vi "Chart with date and time.vi"(11 "Data in":dbl) -> (3 "Waveform Chart":waveform(dbl)(graph))   [LabVIEW 2018]
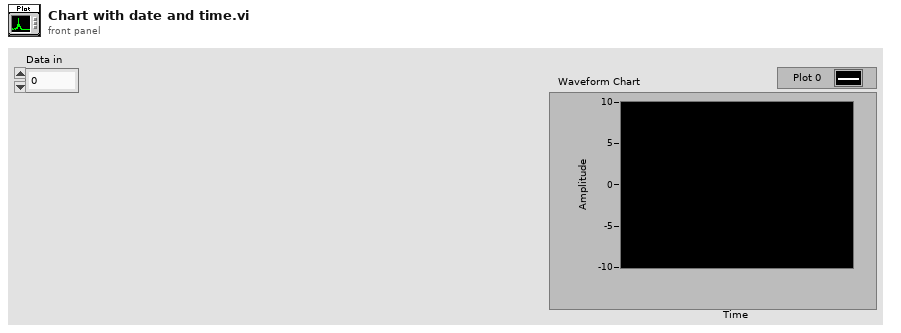
[diagram p1: front panel]
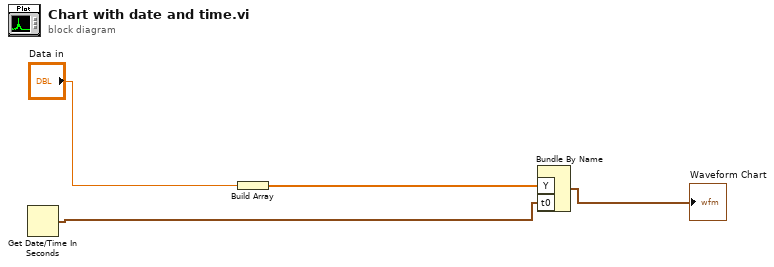
[diagram p0: block diagram]
diagram:
  n1 = Get Date/Time In Seconds() -> (seconds since 1Jan1904=w1:timestamp)
  n2 = Build Array("Data in") -> (w3:dbl[])
  n3 = Bundle By Name("Y"=w3, "t0"=w1) -> (→"Waveform Chart":waveform(dbl))  [unwired: 1 in]
